vi "Preprocess Balloon Data.vi"(8 "error in (no error)":errorcluster, 10 "Output Data File Path":path, 11 "Input Data File Path":path) -> (0 "error out":errorcluster, 3 "Preprocessed Data":dbl[][](array[numeric]))   [LabVIEW 2013]
uses:
  <vilib>/Utility/file.llb/Read From Spreadsheet File (string).vi
  <vilib>/Utility/file.llb/Write To Spreadsheet File (string).vi
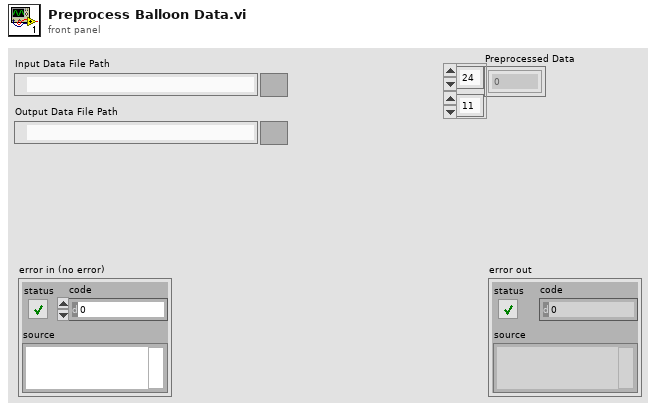
[diagram p1: front panel]
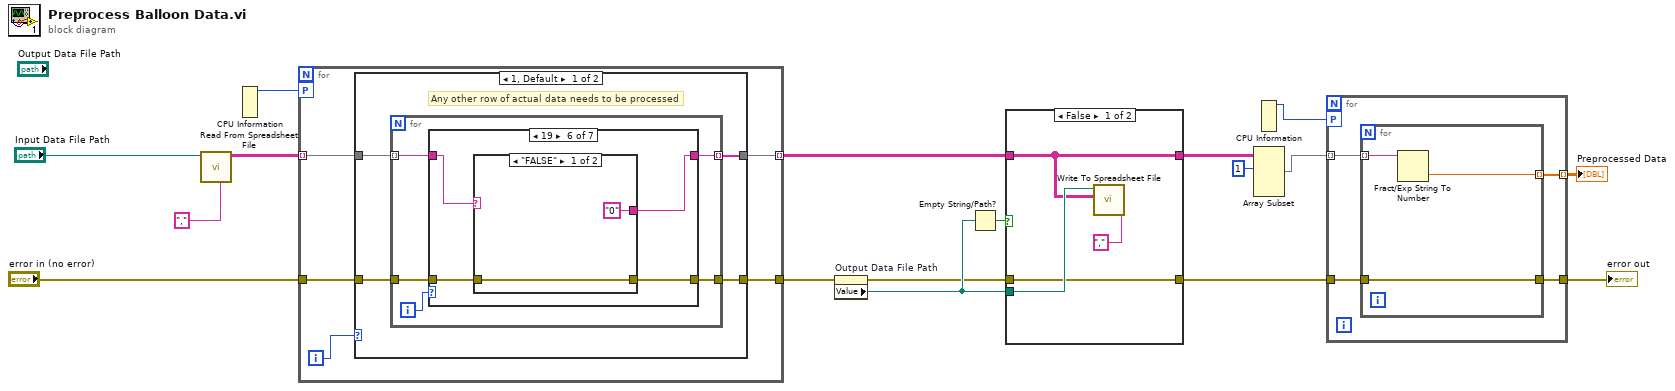
[diagram p0: block diagram]
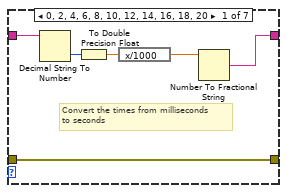
[diagram p3: hidden frame]
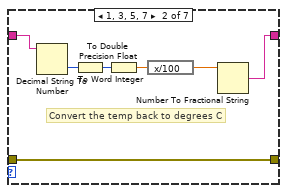
[diagram p4: hidden frame]
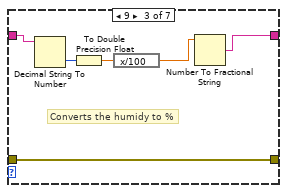
[diagram p5: hidden frame]
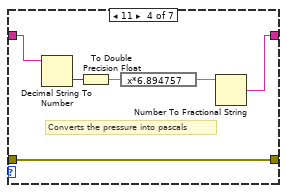
[diagram p6: hidden frame]
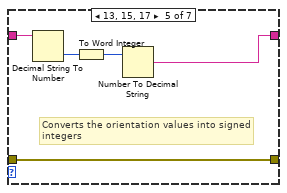
[diagram p7: hidden frame]
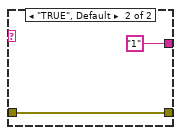
[diagram p8: hidden frame]
diagram:
  n1 = call-poly <vilib>:"Read From Spreadsheet File.vi"("delimiter (\\t)"="," ("delimiter (\\t)"), "file path (dialog if empty)"="Input Data File Path") -> ("all rows"=w15:string[][])  [unwired: 5 in, 4 out]
  n2 = CPU Information() -> (4:w1:i32)  [unwired: 3 out]
  n3 = for {
    tunnel: w15 -> [w21] mode=indexing
    tunnel: [w20] -> w13 mode=indexing
    tunnel: "error in (no error)" -> [w18]
    tunnel: [w19] -> w12
    workers-P: w1 -> [_]
    i -> [w22]
    n4 = case shown="1, Default" w22 {
      tunnel: w21 -> [w26 w73]
      tunnel: [w23 w73] -> w20
      tunnel: w18 -> [w25 w72]
      tunnel: [w24 w72] -> w19
      frame 1, Default {
        # "Any other row of actual data needs to be processed"
        n5 = for {
          tunnel: w26 -> [w28] mode=indexing
          tunnel: w25 -> [w30]
          tunnel: [w29] -> w24
          tunnel: [w27] -> w23 mode=indexing
          i -> [w31]
          n6 = case shown="19" w31 {
            tunnel: w30 -> [w37 w38 w50 w51 w57 w64 w70]
            tunnel: [w37 w38 w50 w51 w57 w63 w70] -> w29
            tunnel: w28 -> [w36 w42 w48 w54 w61 w65 w71]
            tunnel: [w32 w39 w45 w52 w58 w62 w71] -> w27
            frame 0, 2, 4, 6, 8, 10, 12, 14, 16, 18, 20 {
              # "Convert the times from milliseconds\nto seconds"
              n7 = Decimal String To Number(string=w36) -> (number=w35:i32)  [unwired: 2 in, 1 out]
              n8 = To Double Precision Float(number=w35) -> (double precision float=w34:dbl)
              n9 = expression code="x/1000"(w34) -> (w33:dbl)
              n10 = Number To Fractional String(number=w33) -> (F-format string=w32:string)  [unwired: 3 in]
            }
            frame 1, 3, 5, 7 {
              # "Convert the temp back to degrees C"
              n11 = Decimal String To Number(string=w42) -> (number=w43:i32)  [unwired: 2 in, 1 out]
              n12 = To Word Integer(number=w43) -> (16bit integer=w44:i16)
              n13 = To Double Precision Float(number=w44) -> (double precision float=w41:dbl)
              n14 = expression code="x/100"(w41) -> (w40:dbl)
              n15 = Number To Fractional String(number=w40) -> (F-format string=w39:string)  [unwired: 3 in]
            }
            frame 9 {
              # "Converts the humidy to %"
              n16 = Decimal String To Number(string=w48) -> (number=w49:i32)  [unwired: 2 in, 1 out]
              n17 = To Double Precision Float(number=w49) -> (double precision float=w47:dbl)
              n18 = expression code="x/100"(w47) -> (w46:dbl)
              n19 = Number To Fractional String(number=w46) -> (F-format string=w45:string)  [unwired: 3 in]
            }
            frame 11 {
              # "Converts the pressure into pascals"
              n20 = Decimal String To Number(string=w54) -> (number=w56:i32)  [unwired: 2 in, 1 out]
              n21 = To Double Precision Float(number=w56) -> (double precision float=w55:dbl)
              n22 = expression code="x*6.894757"(w55) -> (w53:dbl)
              n23 = Number To Fractional String(number=w53) -> (F-format string=w52:string)  [unwired: 3 in]
            }
            frame 13, 15, 17 {
              # "Converts the orientation values into signed \nintegers"
              n24 = Decimal String To Number(string=w61) -> (number=w60:i32)  [unwired: 2 in, 1 out]
              n25 = To Word Integer(number=w60) -> (16bit integer=w59:i16)
              n26 = Number To Decimal String(number=w59) -> (decimal integer string=w58:string)  [unwired: 1 in]
            }
            frame 19 {
              n27 = case shown="\"FALSE\"" w65 {
                tunnel: w64 -> [w66 w69]
                tunnel: [w66 w69] -> w63
                tunnel: ["0" "1"] -> w62
                frame "FALSE" {
                }
                frame "TRUE", Default {
                }
              }
            }
            frame Default {
              # "Some other value; just pass it through without\nany modifications."
            }
          }
        }
      }
      frame 0 {
        # "This is the first row (just displays the type of data)"
      }
    }
  }
  n28 = property on="Output Data File Path" class="Path"(error in=w12) -> (error out=w9:errorcluster, "Value"=w10:path)  [unwired: 1 in, 1 out]
  n29 = Empty String/Path?(string/path=w10) -> (empty?=w11:bool)
  n30 = case shown="False" w11 {
    tunnel: w13 -> [w74 w79]
    tunnel: w10 -> [w76 _]
    tunnel: [w74 w79] -> w6
    tunnel: w9 -> [w75 w78]
    tunnel: [w75 w78] -> w8
    frame False {
      n31 = call-poly <vilib>:"Write To Spreadsheet File.vi"("delimiter (\\t)"="," ("delimiter (\\t)"), "2D data"=w74, "file path (dialog if empty)"=w76) -> ()  [unwired: 5 in, 1 out]
    }
    frame True {
    }
  }
  n32 = CPU Information() -> (4:w3:i32)  [unwired: 3 out]
  n33 = Array Subset(array=w6, index (row)=1 ("index")) -> (w5:string[][])  [unwired: 3 in]
  n34 = for {
    tunnel: w8 -> [w83]
    tunnel: w5 -> [w81] mode=indexing
    tunnel: [w82] -> w7
    tunnel: [w80] -> w2 mode=indexing
    workers-P: w3 -> [_]
    n35 = for {
      tunnel: w83 -> [w86]
      tunnel: [w86] -> w82
      tunnel: w81 -> [w85] mode=indexing
      tunnel: [w84] -> w80 mode=indexing
      n36 = Fract/Exp String To Number(string=w85) -> (number=w84:dbl)  [unwired: 3 in, 1 out]
    }
  }
  "error out" <- w7
  "Preprocessed Data" <- w2
